vi "ma_SML Filtered Spectrum.vi"(0 "power spectrum":T1 {"spectrum" format="%.2f"; "df" format="%.2f"; "f0" format="%.2f"}, 5 "spectral info":T2 {"window" items=["Rectangle"=0, "Hanning"=1, "Hamming"=2, "Blackman-Harris"=3, "Exact Blackman"=4, "Blackman"=5, "Flat Top"=6, "4 Term B-Harris "=7, "7 Term B-Harris"=8, "Low Sidelobe"=9, "Blackman Nuttall"=11, "Triangle"=30, "Bartlett-Hanning"=31, "Bohman"=32, "Parzen"=33, "Welch"=34, "Kaiser"=60, "Dolph-Chebyshev"=61, "Gaussian"=62]}, 7 "filter power spectrum":T1 {"spectrum" format="%.2f"; "df" format="%.2f"; "f0" format="%.2f"}, 11 "error in (no error)":errorcluster) -> (4 "filtered power spectrum":T1 {"spectrum" format="%.2f"; "df" format="%.2f"; "f0" format="%.2f"}, 15 "error out":errorcluster)   [LabVIEW 2020, in "NI_MAPro.lvlib"]
uses:
  NI_MAPro.lvlib
  ma_sml_Spectrum Cluster (real).ctl
  ma_sml_Spectral Info.ctl
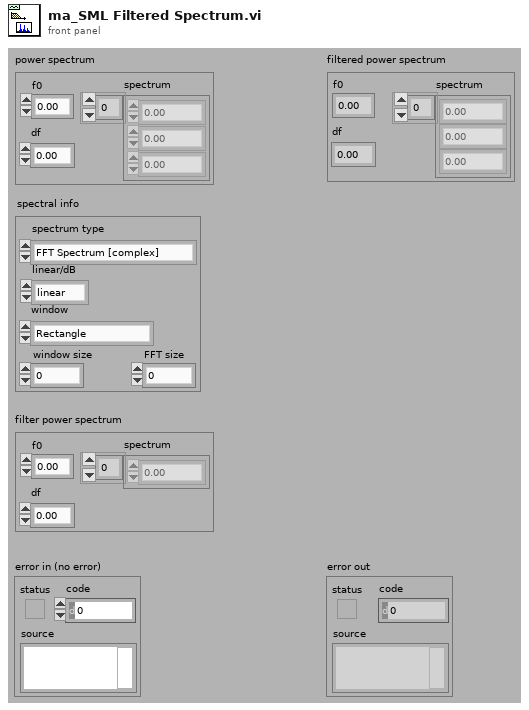
[diagram p1: front panel]
types:
  T1 = typedef "NI_MAPro.lvlib/ma_sml_Spectrum Cluster (real).ctl" = cluster{"f0":dbl, "df":dbl, "spectrum":dbl[]}
  T2 = typedef "NI_MAPro.lvlib/ma_sml_Spectral Info.ctl" = cluster{"spectrum type":enum16{"FFT Spectrum [complex]", "Amplitude [Magnitude]", "Power [Magnitude^2]", "Cross Spectrum [complex]", "Frequency Response [Complex]"}, "linear/dB":enum16{"linear", "dB"}, "window":u16, "window size":i32, "FFT size":i32}
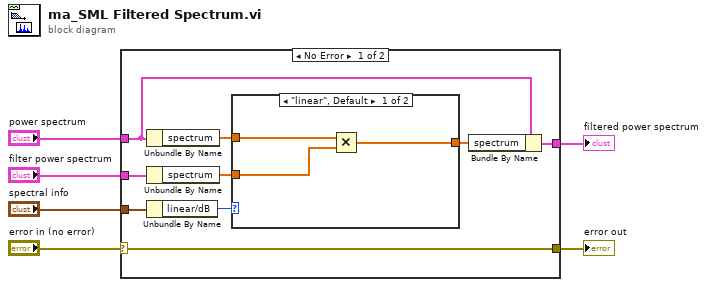
[diagram p0: block diagram]
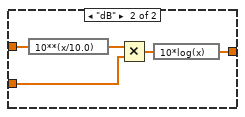
[diagram p2: hidden frame]
diagram:
  n1 = case shown="No Error" "error in (no error)" {
    selector: "error in (no error)" -> [w9 w24]
    tunnel: "spectral info" -> [w12 _]
    tunnel: "power spectrum" -> [w11 _]
    tunnel: [w10 _] -> w4
    tunnel: [w9 w24] -> w2
    tunnel: "filter power spectrum" -> [w8 _]
    frame No Error {
      n2 = Unbundle By Name(w11) -> ("spectrum"=w14:dbl[])
      n3 = Unbundle By Name(w8) -> ("spectrum"=w7:dbl[])
      n4 = Unbundle By Name(w12) -> ("linear/dB"=w13:enum16{"linear", "dB"})
      n5 = case shown="\"linear\", Default" w13 {
        tunnel: w7 -> [w16 w19]
        tunnel: w14 -> [w18 w23]
        tunnel: [w17 w20] -> w15
        frame "linear", Default {
          n6 = Multiply(x=w18, y=w16) -> (x*y=w17:dbl[])
        }
        frame "dB" {
          n7 = expression code="10**(x/10.0)"(w23) -> (w22:dbl[])
          n8 = Multiply(x=w22, y=w19) -> (x*y=w21:dbl[])
          n9 = expression code="10*log(x)"(w21) -> (w20:dbl[])
        }
      }
      n10 = Bundle By Name(cluster=w11, "spectrum"=w15) -> (w10:T1)
    }
    frame Error {
    }
  }
  "filtered power spectrum" <- w4
  "error out" <- w2
